vi "Omron TCP FINS-Write Data(Boolean Element).vi"(8 "error in":errorcluster, 9 "Data":bool, 10 "Write Setting(Boolean Element)":T1={"I/O Memory Address"=130, "Data Address"=0, "Bit Index"=0} {"I/O Memory Address" items=["DM"=130, "CIO"=176, "WR"=177, "HR"=178, "AR"=179, "TIM"=137, "EM"=152]}, 11 "Buffer Data In":T2) -> (0 "error out":errorcluster, 3 "Buffer Data Out":T2)   [LabVIEW 2016]
uses:
  Data Def/Omron TCP FINS-Buffer Data.ctl
  Data Def/Omron TCP FINS-Command Code.ctl
  Data Def/Omron TCP FINS-FINS Command Frame.ctl
  Data Def/Omron TCP FINS-Memory Area Read Data.ctl
  Data Def/Omron TCP FINS-Memory Area Write Data.ctl
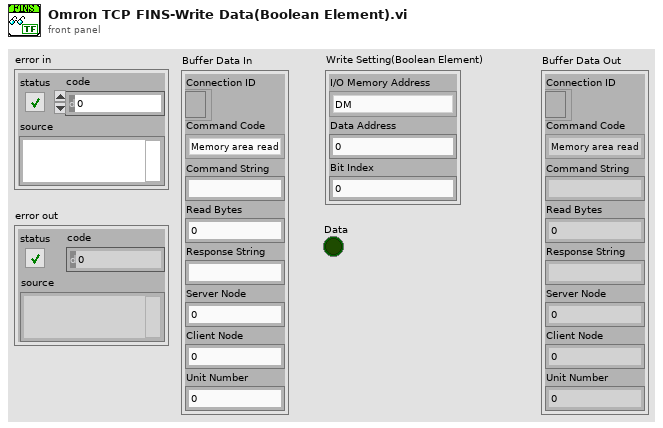
[diagram p1: front panel]
types:
  T1 = cluster{"I/O Memory Address":u8, "Data Address":u16, "Bit Index":i32}
  T2 = typedef "Omron TCP FINS-Buffer Data.ctl" = cluster{"Connection ID":refnum<k5>, "Command Code":T3, "Command String":string, "Read Bytes":i32, "Response String":string, "Server Node":u8, "Client Node":u8, "Unit Number":u8}
  T3 = typedef "Omron TCP FINS-Command Code.ctl" = enum16{"Memory area read", "Memory area write"}
  T4 = typedef "Omron TCP FINS-FINS Command Frame.ctl" = cluster{"Command Code":T3, "Command Data":variant}
  T5 = typedef "Omron TCP FINS-Memory Area Write Data.ctl" = cluster{"I/O Memory Address":u8, "Beginning Address":u16, "Data":i16[]}
  T6 = typedef "Omron TCP FINS-Memory Area Read Data.ctl" = cluster{"I/O Memory Address":u8, "Beginning Address":u16, "No. Of Items":u16}
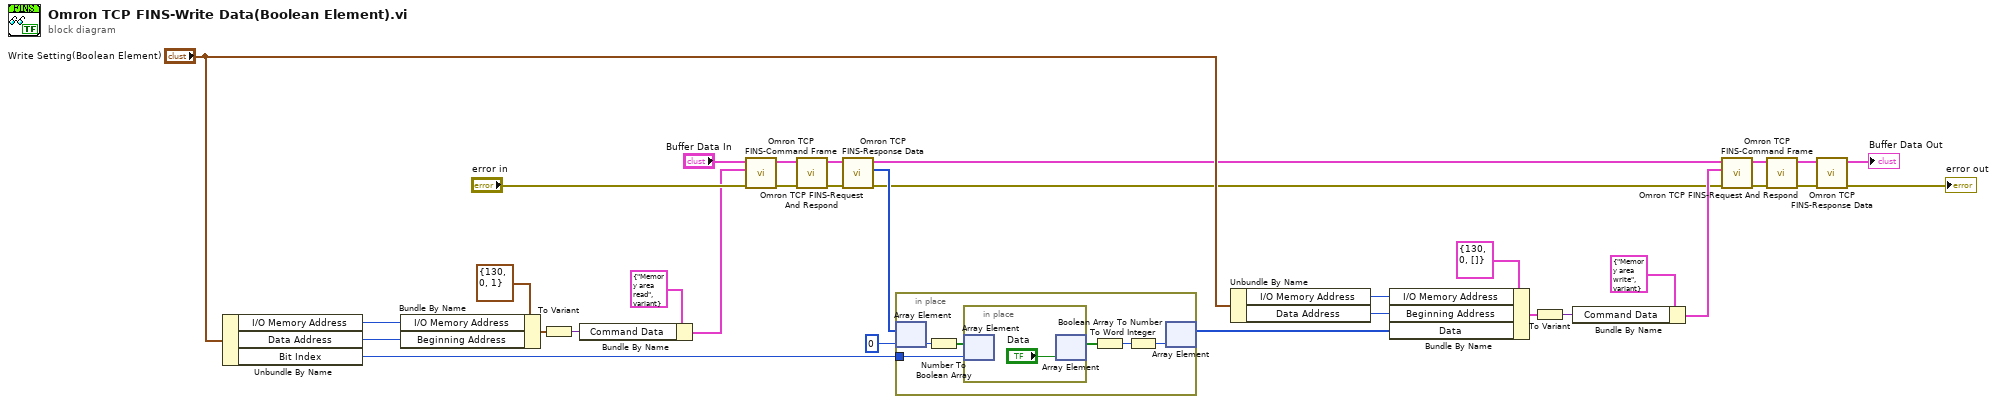
[diagram p0: block diagram]
diagram:
  n1 = Unbundle By Name("Write Setting(Boolean Element)") -> ("I/O Memory Address"=w18:u8, "Data Address"=w17:u16, "Bit Index"=w21:i32)
  n2 = Bundle By Name(cluster=T6 {"I/O Memory Address"=130, "Beginning Address"=0, "No. Of Items"=1} ("Memory Area Read Data"), "I/O Memory Address"=w18, "Beginning Address"=w17) -> (w26:T6)
  n3 = To Variant(anything=w26) -> (Variant=w31:variant)
  n4 = Bundle By Name(cluster=T4 {"Command Code"=enum."Memory area read", "Command Data"=variant} ("FINS Command Frame"), "Command Data"=w31) -> (w29:T4)
  n5 = call "Omron TCP FINS-Command Frame.vi"("error in"="error in", "FINS Command Frame"=w29, "Buffer Data In"="Buffer Data In") -> ("error out"=w27:errorcluster, "Buffer Data Out"=w28:T2)  [unwired: 7 in]
  n6 = call "Omron TCP FINS-Request And Respond.vi"("error in"=w27, "Buffer Data In"=w28) -> ("error out"=w23:errorcluster, "Buffer Data Out"=w24:T2)  [unwired: 8 in]
  n7 = call "Omron TCP FINS-Response Data.vi"("error in"=w23, "Buffer Data In"=w24) -> ("error out"=w3:errorcluster, "Data"=w22:i16[], "Buffer Data Out"=w2:T2)  [unwired: 7 in]
  n8 = in-place {
    in-place-border: w21 -> [w37]
    n9 = in-place-array #1(w22, 0) -> (w39:i16)
    n10 = Number To Boolean Array(number=w39) -> (Boolean array=w38:bool[])
    n11 = in-place {
      n12 = in-place-array #2(w38, w37) -> ()  [unwired: 1 out]
      n13 = in-place-array #2("Data") -> (w36:bool[])  [unwired: 1 out]
    }
    n14 = Boolean Array To Number(Boolean array=w36) -> (number=w35:u32)
    n15 = To Word Integer(number=w35) -> (16bit integer=w34:i16)
    n16 = in-place-array #1(w34) -> (w12:i16[])  [unwired: 1 out]
  }
  n17 = Unbundle By Name("Write Setting(Boolean Element)") -> ("I/O Memory Address"=w14:u8, "Data Address"=w13:u16)
  n18 = Bundle By Name(cluster=T5 {"I/O Memory Address"=130, "Beginning Address"=0, "Data"=[]} ("Memory Area Write Data"), "I/O Memory Address"=w14, "Beginning Address"=w13, "Data"=w12) -> (w16:T5)
  n19 = To Variant(anything=w16) -> (Variant=w11:variant)
  n20 = Bundle By Name(cluster=T4 {"Command Code"=enum."Memory area write", "Command Data"=variant} ("FINS Command Frame"), "Command Data"=w11) -> (w4:T4)
  n21 = call "Omron TCP FINS-Command Frame.vi"("error in"=w3, "FINS Command Frame"=w4, "Buffer Data In"=w2) -> ("error out"=w5:errorcluster, "Buffer Data Out"=w6:T2)  [unwired: 7 in]
  n22 = call "Omron TCP FINS-Request And Respond.vi"("error in"=w5, "Buffer Data In"=w6) -> ("error out"=w9:errorcluster, "Buffer Data Out"=w20:T2)  [unwired: 8 in]
  n23 = call "Omron TCP FINS-Response Data.vi"("error in"=w9, "Buffer Data In"=w20) -> ("error out"=→"error out":errorcluster, "Buffer Data Out"=→"Buffer Data Out":T2)  [unwired: 7 in, 1 out]
